vi "Joystick Deadband.vi"(7 "Deadband":dbl(knob) scale=0.0..0.5, 9 "Y in":dbl(slide) scale=-1.0..1.0, 10 "X in":dbl(slide) scale=-1.0..1.0) -> (1 "Y out":dbl(slide) scale=-1.0..1.0, 2 "X out":dbl(slide) scale=-1.0..1.0)   [LabVIEW 2013, in "XBoxController.lvclass"]
uses:
  XBoxController.lvclass
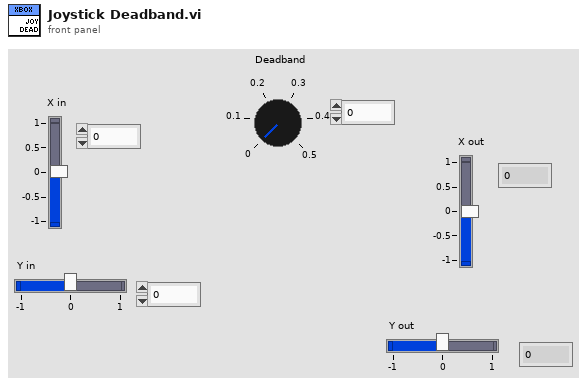
[diagram p1: front panel]
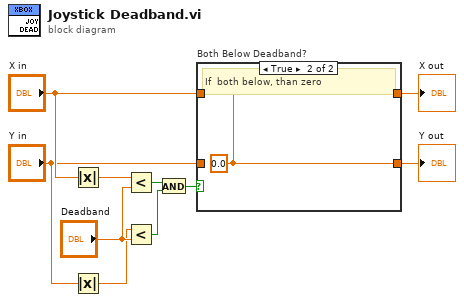
[diagram p0: block diagram]
diagram:
  n1 = Absolute Value(x="X in") -> (abs(x)=w2:dbl)
  n2 = Absolute Value(x="Y in") -> (abs(x)=w1:dbl)
  n3 = Less?(x=w2, y="Deadband") -> (x < y?=w9:bool)
  n4 = Less?(x=w1, y="Deadband") -> (x < y?=w8:bool)
  n5 = And(x=w9, y=w8) -> (x .and. y?=w7:bool)
  n6 = case "Both Below Deadband?" shown="True" w7 {
    tunnel: "X in" -> [w12 _]
    tunnel: [w12 w13] -> w5
    tunnel: "Y in" -> [w11 _]
    tunnel: [w11 w13] -> w3
    frame False {
      # "Not both below so ignore deadband"
    }
    frame True {
      w13 = 0.0 ("X in")
      # "If  both below, than zero"
    }
  }
  "X out" <- w5
  "Y out" <- w3
